vi "Control Refs.vi"(8 "error in (no error)":errorcluster, 11 "Plugin Splash in":refnum<class "Plugin Splash.lvclass">) -> (0 "error out":errorcluster, 3 "Plugin Splash out":refnum<class "Plugin Splash.lvclass">)   [LabVIEW 2020, in "Volatus.lvlib" / "Plugin Splash.lvclass"]
uses:
  Plugin Splash.lvclass
  Plugin Splash.lvclass/Plugin Splash.ctl
  Refs.ctl
  lv-builder/Builder Core/Builder Core.lvlib
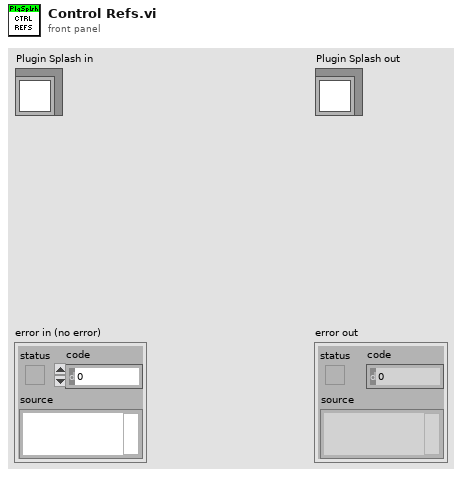
[diagram p1: front panel]
types:
  T1 = typedef "Volatus.lvlib/Plugin Splash.lvclass/Refs.ctl" = cluster{"Status":refnum<vi>, "Version":refnum<vi>}
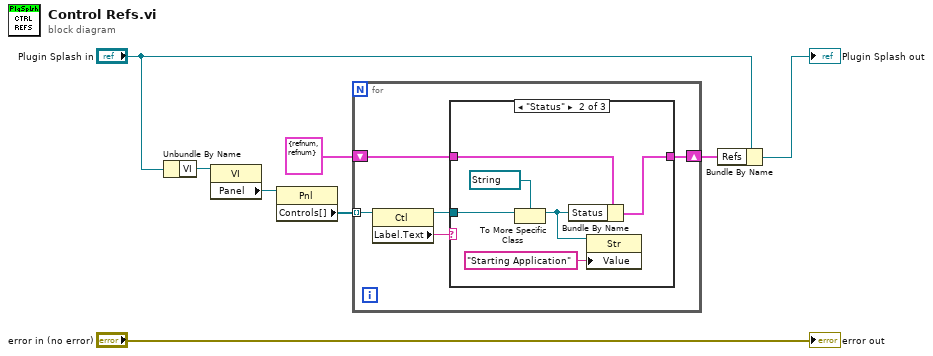
[diagram p0: block diagram]
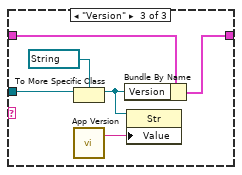
[diagram p3: hidden frame]
diagram:
  n1 = Unbundle By Name("Plugin Splash in") -> ("VI"=w6:refnum<vi>)
  n2 = property class="VI"(reference=w6) -> ("Panel"=w5:refnum<vi>)  [unwired: 1 in, 2 out]
  n3 = property class="Pnl"(reference=w5) -> ("Controls[]"=w4:refnum<vi>[])  [unwired: 1 in, 2 out]
  n4 = for {
    tunnel: w4 -> [w13] mode=indexing
    shift-right: [w11] -> w1
    shift-left: T1 {"Status"=refnum, "Version"=refnum} ("Refs") -> [w10]
    n5 = property class="Ctl"(reference=w13) -> (reference out=w9:refnum<vi>, "Label.Text"=w12:string)  [unwired: 1 in, 1 out]
    n6 = case shown="\"Status\"" w12 {
      tunnel: [w14 w19 w25] -> w11
      tunnel: w10 -> [w14 w20 w26]
      tunnel: w9 -> [_ w18 w24]
      frame Default {
      }
      frame "Status" {
        n7 = To More Specific Class(target class=refnum<vi> refnum ("Status"), reference=w18) -> (specific class reference=w16:refnum<vi>)  [unwired: 1 in, 1 out]
        n8 = Bundle By Name(cluster=w20, "Status"=w16) -> (w19:T1)
        n9 = property class="Str"(reference=w16, "Value"="Starting Application") -> ()  [unwired: 1 in, 2 out]
      }
      frame "Version" {
        n10 = To More Specific Class(target class=refnum<vi> refnum ("Status"), reference=w24) -> (specific class reference=w22:refnum<vi>)  [unwired: 1 in, 1 out]
        n11 = call "App Version.vi"() -> ("App Version String"=w21:string)  [unwired: 7 in]
        n12 = Bundle By Name(cluster=w26, "Version"=w22) -> (w25:T1)
        n13 = property class="Str"(reference=w22, "Value"=w21) -> ()  [unwired: 1 in, 2 out]
      }
    }
  }
  n14 = Bundle By Name(cluster="Plugin Splash in", "Refs"=w1) -> (→"Plugin Splash out":refnum<class "Plugin Splash.lvclass">)
  "error out" <- "error in (no error)"
